vi "TCP Errors - Full List.vi"(11 "Include Expected Timeouts?":bool) -> (3 "TCP Errors to Clear":i32[](array[numeric])=[56, 66, 62, 1])   [LabVIEW 2013, in "TS.lvlib"]
uses:
  TS.lvlib
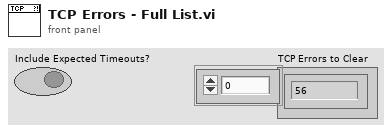
[diagram p1: front panel]
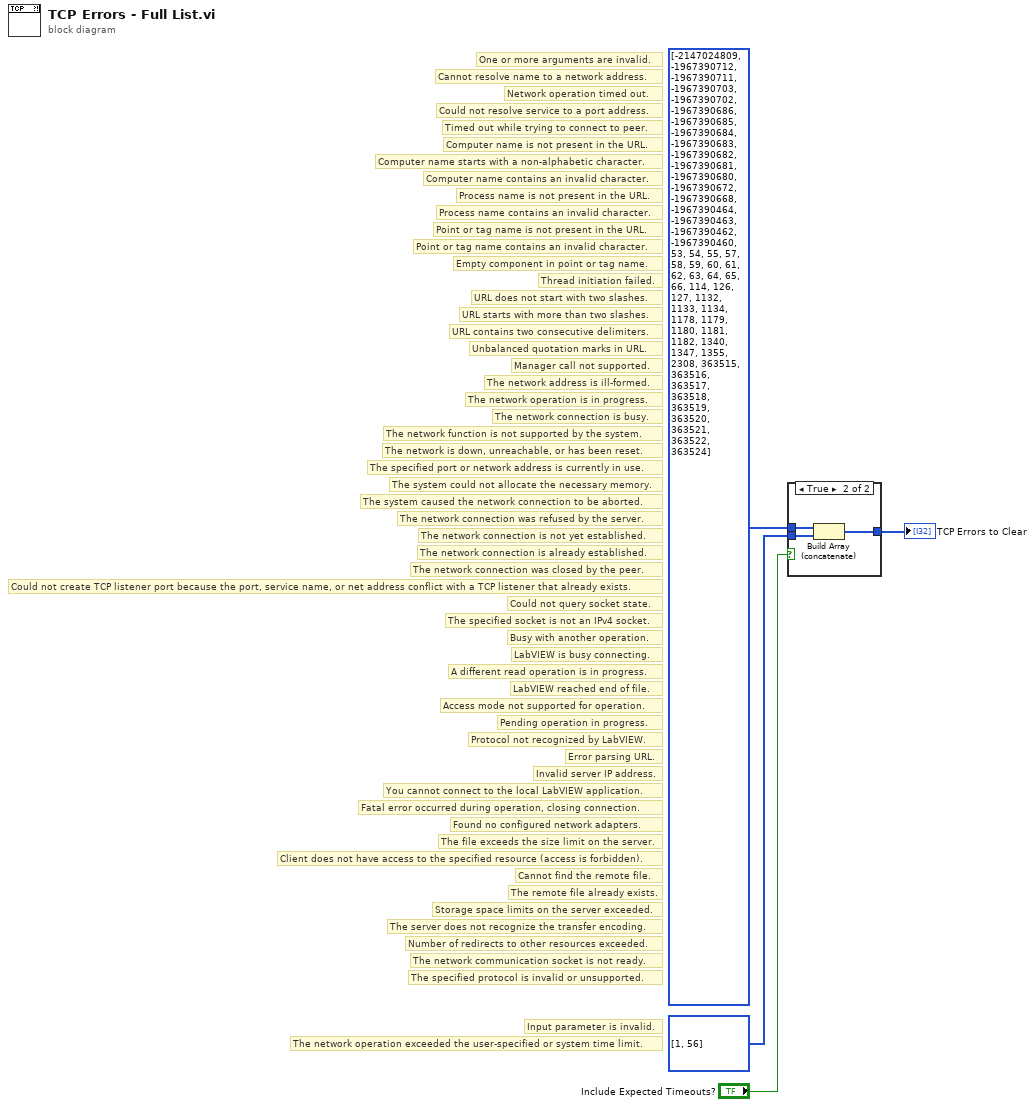
[diagram p0: block diagram]
diagram:
  # "Input parameter is invalid."
  # "The specified protocol is invalid or unsupported."
  # "The network communication socket is not ready."
  # "Number of redirects to other resources exceeded."
  # "The server does not recognize the transfer encoding."
  # "Storage space limits on the server exceeded."
  # "The remote file already exists."
  # "Cannot find the remote file."
  # "Client does not have access to the specified resource (access is forbidden)."
  # "The file exceeds the size limit on the server."
  # "Found no configured network adapters."
  # "Fatal error occurred during operation, closing connection."
  # "You cannot connect to the local LabVIEW application."
  # "Invalid server IP address."
  # "Error parsing URL."
  # "Protocol not recognized by LabVIEW."
  # "Pending operation in progress."
  # "Access mode not supported for operation."
  # "LabVIEW reached end of file."
  # "A different read operation is in progress."
  # "LabVIEW is busy connecting."
  # "Busy with another operation."
  # "The specified socket is not an IPv4 socket."
  # "Could not query socket state."
  # "Could not create TCP listener port because the port, service name, or net address conflict with a TCP listener that already exists."
  # "The network connection was closed by the peer."
  # "The network connection is already established."
  # "The network connection is not yet established."
  # "The network connection was refused by the server."
  # "The system caused the network connection to be aborted."
  # "The system could not allocate the necessary memory."
  # "The specified port or network address is currently in use."
  # "The network is down, unreachable, or has been reset."
  # "The network function is not supported by the system."
  # "The network connection is busy."
  # "The network operation exceeded the user-specified or system time limit."
  # "The network operation is in progress."
  # "The network address is ill-formed."
  # "Manager call not supported."
  # "Unbalanced quotation marks in URL."
  # "URL contains two consecutive delimiters."
  # "URL starts with more than two slashes."
  # "URL does not start with two slashes."
  # "Thread initiation failed."
  # "Empty component in point or tag name."
  # "Point or tag name contains an invalid character."
  # "Point or tag name is not present in the URL."
  # "Process name contains an invalid character."
  # "Process name is not present in the URL."
  # "Computer name contains an invalid character."
  # "Computer name starts with a non-alphabetic character."
  # "Computer name is not present in the URL."
  # "Timed out while trying to connect to peer."
  # "Could not resolve service to a port address."
  # "Network operation timed out."
  # "Cannot resolve name to a network address."
  # "One or more arguments are invalid."
  n1 = case shown="True" "Include Expected Timeouts?" {
    tunnel: i32[] [-2147024809, -1967390712, -1967390711, -1967390703, -1967390702, -1967390686, -1967390685, -1967390684, -1967390683, -1967390682, -1967390681, -1967390680, -1967390672, -1967390668, -1967390464, -1967390463, -1967390462, -1967390460, 53, 54, 55, 57, 58, 59, 60, 61, 62, 63, 64, 65, 66, 114, 126, 127, 1132, 1133, 1134, 1178, 1179, 1180, 1181, 1182, 1340, 1347, 1355, 2308, 363515, 363516, 363517, 363518, 363519, 363520, 363521, 363522, 363524] ("Errors to Clear") -> [w5 w8]
    tunnel: i32[] [1, 56] ("Errors to Clear") -> [_ w7]
    tunnel: [w5 w6] -> w1
    frame False {
    }
    frame True {
      n2 = Build Array (concatenate)(w8, w7) -> (w6:i32[])
    }
  }
  "TCP Errors to Clear" <- w1
